vi "PrepareMap.vi"(7 "Map":refnum<vi>, 10 "All Lines out":T1) -> (2 "Array":cluster{cluster{"X":dbl, "Z":dbl}[]}[](array[cluster]))   [LabVIEW 2014]
uses:
  Libraries/Map Data Folder/All-Lines.ctl
  Libraries/Map Data Folder/LineCluster.ctl
  Libraries/Map Data Folder/LineConnection.ctl
  Libraries/Map Data Folder/Map Data.lvlib
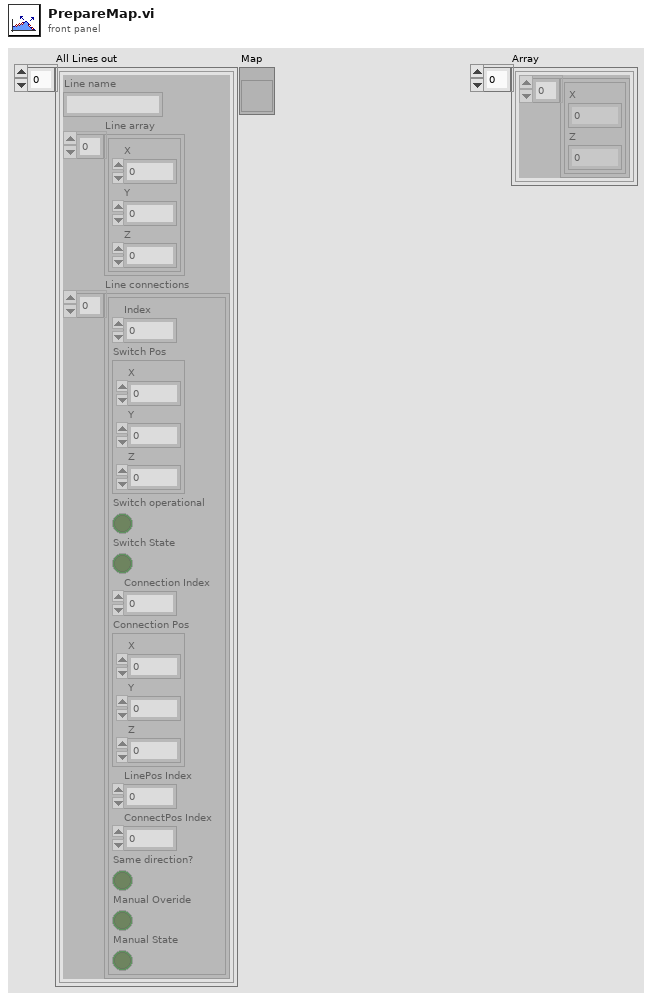
[diagram p1: front panel]
types:
  T1 = typedef "Map Data.lvlib/All-Lines.ctl" = T2[]
  T2 = typedef "Map Data.lvlib/LineCluster.ctl" = cluster{"Line name":string, "Line array":cluster{"X":dbl, "Y":dbl, "Z":dbl}[], "Line connections":T3[]}
  T3 = typedef "Map Data.lvlib/LineConnection.ctl" = cluster{"Index":i32, "Switch Pos":cluster{"X":dbl, "Y":dbl, "Z":dbl}, "Switch operational":bool, "Switch State":bool, "Connection Index":i32, "Connection Pos":cluster{"X":dbl, "Y":dbl, "Z":dbl}, "LinePos Index":i32, "ConnectPos Index":i32, "Same direction?":bool, "Manual Overide":bool, "Manual State":bool}
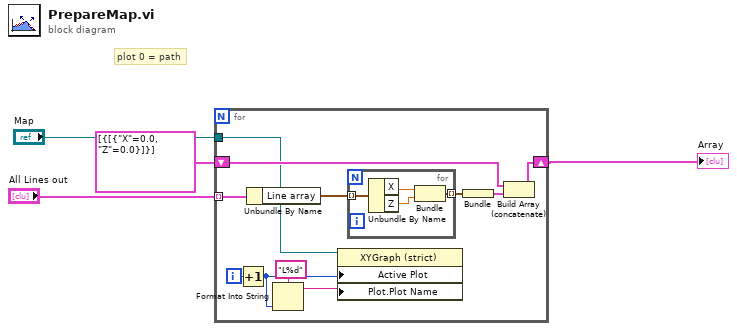
[diagram p0: block diagram]
diagram:
  # "plot 0 = path"
  n1 = for {
    tunnel: "All Lines out" -> [w13] mode=indexing
    shift-right: [w11] -> w1
    shift-left: cluster{cluster{"X":dbl, "Z":dbl}[]}[] [{[{"X"=0.0, "Z"=0.0}]}] -> [w10]
    tunnel: "Map" -> [w9]
    i -> [w7]
    n2 = Increment(x=w7) -> (x+1=w5:i32)
    n3 = Unbundle By Name(w13) -> ("Line array"=w14:cluster{"X":dbl, "Y":dbl, "Z":dbl}[])
    n4 = Format Into String(format string="L%d", w5) -> (resulting string=w6:string)  [unwired: 2 in, 1 out]
    n5 = property on="Property Node" class="XYGraph (strict)"(reference=w9, "Active Plot"=w5, "Plot.Plot Name"=w6) -> ()  [unwired: 1 in, 2 out]
    n6 = for {
      tunnel: w14 -> [w19] mode=indexing
      tunnel: [w16] -> w15 mode=indexing
      n7 = Unbundle By Name(w19) -> ("X"=w18:dbl, "Z"=w17:dbl)
      n8 = Bundle("X"=w18, "Z"=w17) -> (w16:cluster{"X":dbl, "Z":dbl})  [unwired: 1 in]
    }
    n9 = Bundle(w15) -> (w12:cluster{cluster{"X":dbl, "Z":dbl}[]})  [unwired: 1 in]
    n10 = Build Array (concatenate)(w10, w12) -> (w11:cluster{cluster{"X":dbl, "Z":dbl}[]}[])
  }
  "Array" <- w1
